vi "Cascade MEMS Only Header Ver1.0.vi"(8 "Error In":errorcluster, 11 "Measurement Header":string[](array[string])=["CN_0(fF)", "C1_min(fF)", "CN_1(fF)", "C1_max(fF)", "CN_2(fF)", "C2_min(fF)", "CN_3(fF)", "C2_max(fF)", "CN_4(fF)", "C3_min(fF)", "CN_5(fF)", "C3_max(fF)", "CN_6(fF)", "C123_min(fF)", "CN_7(fF)", "C123_max(fF)", "CN_8(fF)", "Delta_C1(fF)", "Delta_C2(fF)", "Delta_C3(fF)", "Delta_C123(fF)", "Delta_C1(%)", "Delta_C2(%)", "Delta_C3(%)", "Delta_C123(%)"]) -> (0 "Error Out":errorcluster, 3 "Name Calculated Header":string[](array[string]))   [LabVIEW 2017]
panel:
  in  "Measurement VPI Header":string[](array[string])=["VPI_Voltage(V)", "VPI_C1_max(fF)", "VPI_CN_1(fF)", "VPI_C2_max(fF)", "VPI_CN_2(fF)", "VPI_C3_max(fF)", "VPI_CN_3(fF)", "VPI_C123_max(fF)", "VPI_CN_4(fF)"]
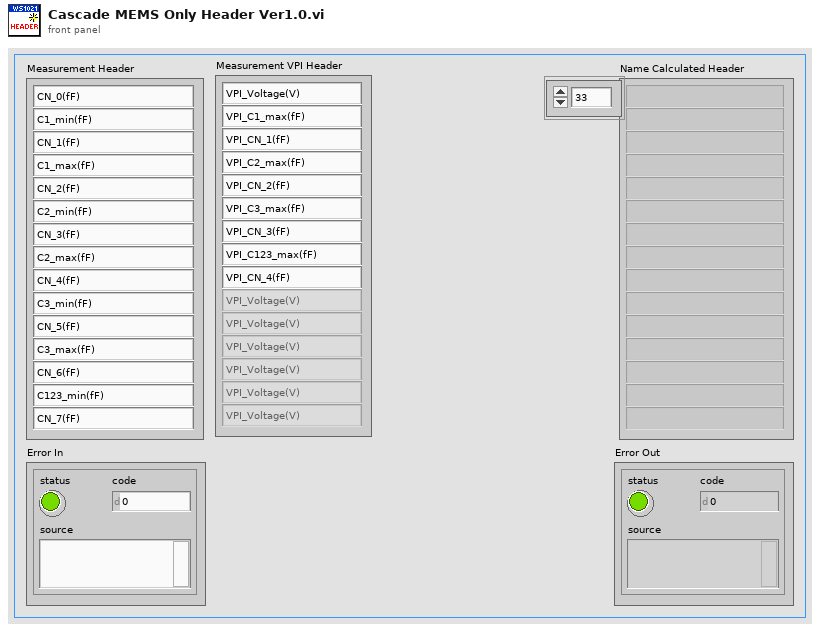
[diagram p1: front panel]
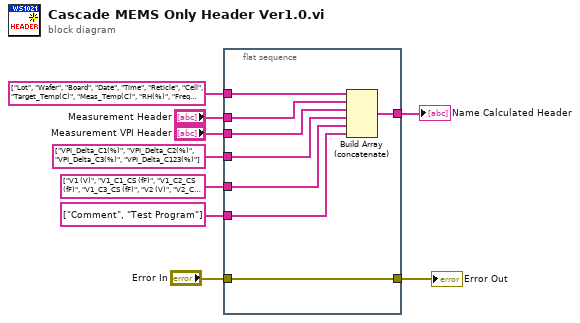
[diagram p0: block diagram]
diagram:
  n1 = flat-sequence {
    tunnel: "Error In" -> [w17]
    tunnel: [w17] -> w9
    tunnel: string[] ["Lot", "Wafer", "Board", "Date", "Time", "Reticle", "Cell", "Target_Temp(C)", "Meas_Temp(C)", "RH(%)", "Freq (KHz)", "Stress_V(V)", "Stress_Beams", "Duty Cycle(%)", "Stress(Min/Num)"] -> [w16]
    tunnel: "Measurement Header" -> [w15]
    tunnel: [w14] -> w6
    tunnel: "Measurement VPI Header" -> [w13]
    tunnel: string[] ["Comment", "Test Program"] -> [w11]
    tunnel: string[] ["VPI_Delta_C1(%)", "VPI_Delta_C2(%)", "VPI_Delta_C3(%)", "VPI_Delta_C123(%)"] -> [w12]
    tunnel: string[] ["V1 (V)", "V1_C1_CS (fF)", "V1_C2_CS (fF)", "V1_C3_CS (fF)", "V2 (V)", "V2_C1_CS (fF)", "V2_C2_CS (fF)", "V2_C3_CS (fF)", "V3 (V)", "V3_C1_CS (fF)", "V3_C2_CS (fF)", "V3_C3_CS (fF)", "VCmin_C1(V)", "VCmin_C2(V)", "VCmin_C3(V)"] -> [w10]
    frame #0 {
      n2 = Build Array (concatenate)(w16, w15, w13, w12, w10, w11) -> (w14:string[])
    }
  }
  "Name Calculated Header" <- w6
  "Error Out" <- w9
